vi "FricModelParam.vi"() -> (3 "FricModelParam":T1(array[cluster]))   [LabVIEW 2017]
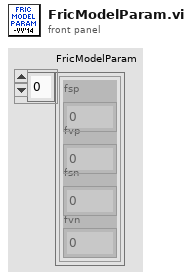
[diagram p1: front panel]
types:
  T1 = cluster{"fsp":dbl, "fvp":dbl, "fsn":dbl, "fvn":dbl}[]
  T2 = cluster{"[0]":dbl, "[1]":dbl, "[2]":dbl, "[3]":dbl}
  T3 = cluster{"[0]":dbl, "[1]":dbl, "[2]":dbl, "[3]":dbl}[]
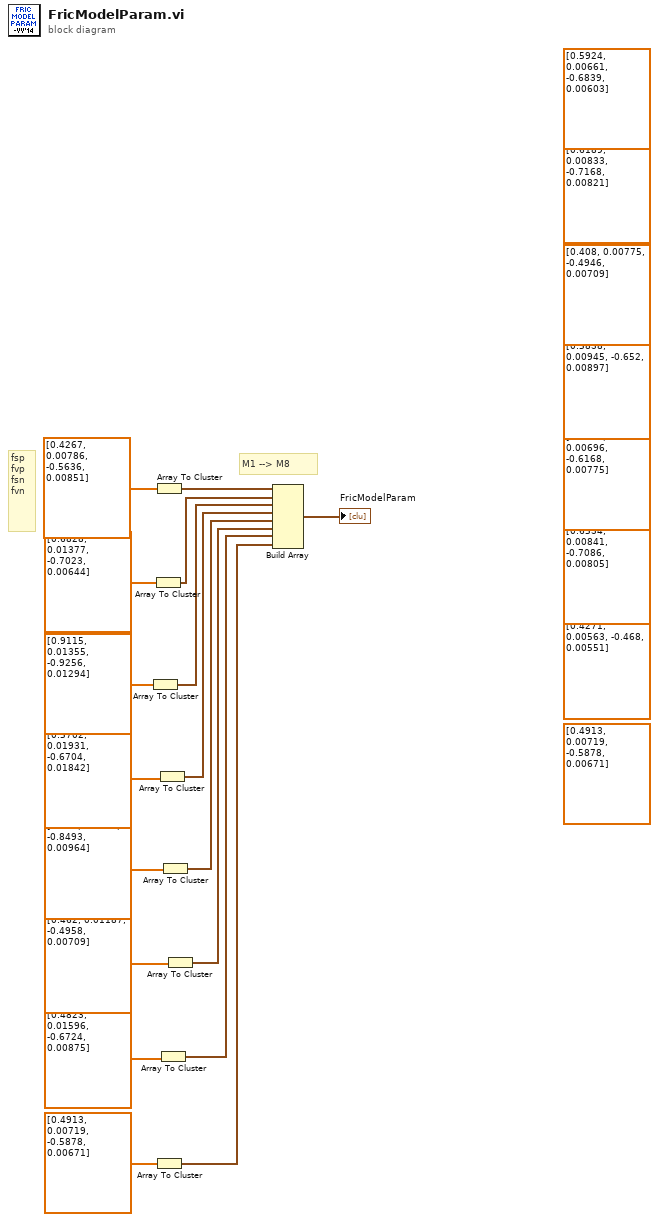
[diagram p0: block diagram]
diagram:
  (unwired) dbl[] [0.4913, 0.00719, -0.5878, 0.00671]
  (unwired) dbl[] [0.4271, 0.00563, -0.468, 0.00551]
  (unwired) dbl[] [0.6534, 0.00841, -0.7086, 0.00805]
  (unwired) dbl[] [0.6074, 0.00696, -0.6168, 0.00775]
  (unwired) dbl[] [0.5838, 0.00945, -0.652, 0.00897]
  (unwired) dbl[] [0.408, 0.00775, -0.4946, 0.00709]
  (unwired) dbl[] [0.6189, 0.00833, -0.7168, 0.00821]
  (unwired) dbl[] [0.5924, 0.00661, -0.6839, 0.00603]
  # "M1 --> M8"
  # "fsp\nfvp\nfsn\nfvn"
  n1 = Array To Cluster(array=dbl[] [0.9115, 0.01355, -0.9256, 0.01294]) -> (cluster=w12:T2)
  n2 = Array To Cluster(array=dbl[] [0.6828, 0.01377, -0.7023, 0.00644]) -> (cluster=w11:T2)
  n3 = Array To Cluster(array=dbl[] [0.4267, 0.00786, -0.5636, 0.00851]) -> (cluster=w10:T2)
  n4 = Array To Cluster(array=dbl[] [0.4913, 0.00719, -0.5878, 0.00671]) -> (cluster=w8:T2)
  n5 = Array To Cluster(array=dbl[] [0.5702, 0.01931, -0.6704, 0.01842]) -> (cluster=w13:T2)
  n6 = Array To Cluster(array=dbl[] [0.4823, 0.01596, -0.6724, 0.00875]) -> (cluster=w16:T2)
  n7 = Array To Cluster(array=dbl[] [0.968, 0.0143, -0.8493, 0.00964]) -> (cluster=w14:T2)
  n8 = Array To Cluster(array=dbl[] [0.462, 0.01187, -0.4958, 0.00709]) -> (cluster=w15:T2)
  n9 = Build Array(w10, w11, w12, w13, w14, w15, w16, w8) -> (→"FricModelParam":T3)
